vi "Obtain Request Events.vi"(8 "error in":errorcluster, 10 "Create New? (F)":bool) -> (0 "error out":errorcluster, 2 "DemoData Generator Request Events":T1)   [LabVIEW 2016, in "DemoData Generator.lvlib"]
doc: "This VI Obtains/Creates the Requests events that will be used for other modules to communicate with the module that owns this VI. These Requests events will be accessed only via Public API methods for this module.\n\n<b>NOTE</b>: The contents of this VI are automatically generated and modified by the <b>Tools > DQMH Consortium > DQMH</b> utilities. Consider using those utilities instead of making your own modifications to this VI.\n_____\nBased on DQMH Project Template 7.0.0.1280."
uses:
  DemoData Generator.lvlib
  Request Events--cluster.ctl
  Stop Argument--cluster.ctl
  Show Panel Argument--cluster.ctl
  Hide Panel Argument--cluster.ctl
  Get Module Execution Status Argument--cluster.ctl
  Show Diagram Argument--cluster.ctl
  Wake-Up Data Reader Argument--cluster.ctl
  Sleep Data Reader Argument--cluster.ctl
  Start Demo Data Argument--cluster.ctl
  Stop Demo Data Argument--cluster.ctl
panel:
  # "NOTE: The contents of this VI are automatically generated and modified by the Tools > DQMH Consortium > DQMH utilities. Consider using those utilities instead of making your own modifications to this VI."
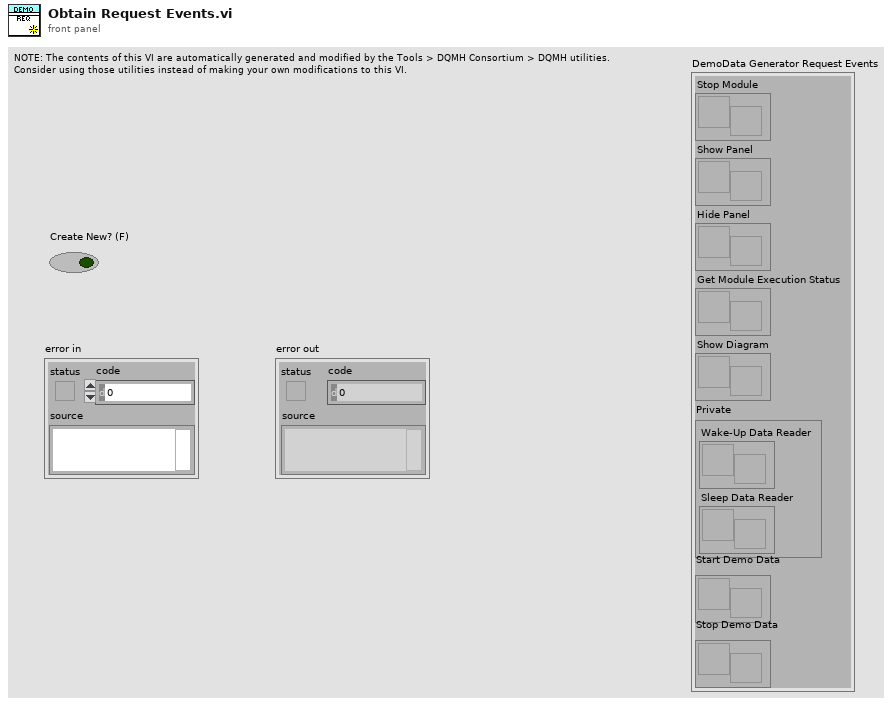
[diagram p1: front panel]
types:
  T1 = typedef "DemoData Generator.lvlib/Request Events--cluster.ctl" = cluster{"Stop Module":refnum<user-event>, "Show Panel":refnum<user-event>, "Hide Panel":refnum<user-event>, "Get Module Execution Status":refnum<user-event>, "Show Diagram":refnum<user-event>, "Private":cluster{"Wake-Up Data Reader":refnum<user-event>, "Sleep Data Reader":refnum<user-event>}, "Start Demo Data":refnum<user-event>, "Stop Demo Data":refnum<user-event>}
  T2 = typedef "DemoData Generator.lvlib/Stop Demo Data Argument--cluster.ctl" = cluster{"Boolean":bool}
  T3 = typedef "DemoData Generator.lvlib/Start Demo Data Argument--cluster.ctl" = cluster{"Boolean":bool}
  T4 = typedef "DemoData Generator.lvlib/Sleep Data Reader Argument--cluster.ctl" = cluster{"Boolean":bool}
  T5 = typedef "DemoData Generator.lvlib/Wake-Up Data Reader Argument--cluster.ctl" = cluster{"Boolean":bool, "Data File.file path":path}
  T6 = typedef "DemoData Generator.lvlib/Hide Panel Argument--cluster.ctl" = cluster{"Hide Panel?":bool}
  T7 = typedef "DemoData Generator.lvlib/Show Panel Argument--cluster.ctl" = cluster{"Show Panel?":bool}
  T8 = typedef "DemoData Generator.lvlib/Show Diagram Argument--cluster.ctl" = cluster{"Debug?":bool}
  T9 = typedef "DemoData Generator.lvlib/Get Module Execution Status Argument--cluster.ctl" = cluster{"Running?":bool}
  T10 = typedef "DemoData Generator.lvlib/Stop Argument--cluster.ctl" = cluster{"Origin":string, "Exit via Stop Module Req?":bool, "Wait for Module to stop?":bool}
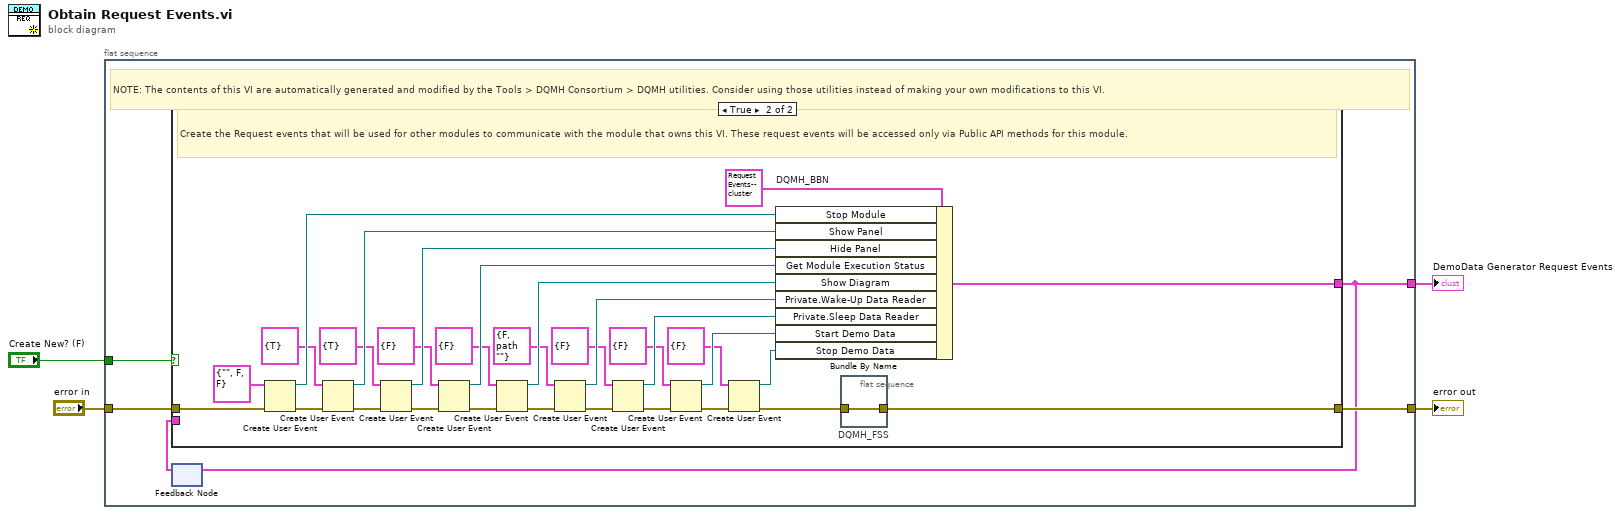
[diagram p0: block diagram]
diagram:
  n1 = flat-sequence {
    tunnel: [w9] -> w4
    tunnel: "error in" -> [w8]
    tunnel: [w6] -> w2
    tunnel: "Create New? (F)" -> [w5]
    frame #0 {
      # "NOTE: The contents of this VI are automatically generated and modified by the Tools > DQMH Consortium > DQMH utilities. Consider using those utilities instead of making your own modifications to this VI."
      n2 = feedback #1() -> (w7:T1)  [unwired: 1 in]
      n3 = case shown="True" w5 {
        tunnel: [w10 w32] -> w9
        tunnel: w8 -> [w10 w42]
        tunnel: [w11 w39] -> w6
        tunnel: w7 -> [w11 _]
        frame False {
          # "Obtain the Request events that were created in a previous call to this VI."
        }
        frame True {
          # "Create the Request events that will be used for other modules to communicate with the module that owns this VI. These request events will be accessed only via Public API methods for this module."
          n4 = Create User Event(user event datatype=T10 {"Origin"="", "Exit via Stop Module Req?"=FALSE, "Wait for Module to stop?"=FALSE} ("Stop Argument"), error in=w42) -> (user event=w40:refnum<user-event>, error out=w37:errorcluster)
          n5 = Create User Event(user event datatype=T7 {"Show Panel?"=TRUE} ("Show Panel Argument"), error in=w37) -> (user event=w36:refnum<user-event>, error out=w35:errorcluster)
          n6 = Create User Event(user event datatype=T6 {"Hide Panel?"=TRUE} ("Hide Panel Argument"), error in=w35) -> (user event=w34:refnum<user-event>, error out=w33:errorcluster)
          n7 = Create User Event(user event datatype=T9 {"Running?"=FALSE} ("Get Module Execution Status Argument"), error in=w33) -> (user event=w30:refnum<user-event>, error out=w31:errorcluster)
          n8 = Create User Event(user event datatype=T8 {"Debug?"=FALSE} ("Show Diagram Argument"), error in=w31) -> (user event=w27:refnum<user-event>, error out=w28:errorcluster)
          n9 = Create User Event(user event datatype=T5 {"Boolean"=FALSE, "Data File.file path"=path ""} ("Wake-Up Data Reader Argument"), error in=w28) -> (user event=w22:refnum<user-event>, error out=w23:errorcluster)
          n10 = Create User Event(user event datatype=T4 {"Boolean"=FALSE} ("Sleep Data Reader Argument"), error in=w23) -> (user event=w19:refnum<user-event>, error out=w20:errorcluster)
          n11 = Create User Event(user event datatype=T3 {"Boolean"=FALSE} ("Start Demo Data Argument"), error in=w20) -> (user event=w16:refnum<user-event>, error out=w17:errorcluster)
          n12 = Create User Event(user event datatype=T2 {"Boolean"=FALSE} ("Stop Demo Data Argument"), error in=w17) -> (user event=w13:refnum<user-event>, error out=w14:errorcluster)
          n13 = Bundle By Name "DQMH_BBN"(cluster=T1 {"Stop Module"=refnum, "Show Panel"=refnum, "Hide Panel"=refnum, "Get Module Execution Status"=refnum, "Show Diagram"=refnum, "Private"={"Wake-Up Data Reader"=refnum, "Sleep Data Reader"=refnum}, "Start Demo Data"=refnum, "Stop Demo Data"=refnum} ("output cluster"), "Stop Module"=w40, "Show Panel"=w36, "Hide Panel"=w34, "Get Module Execution Status"=w30, "Show Diagram"=w27, "Private.Wake-Up Data Reader"=w22, "Private.Sleep Data Reader"=w19, "Start Demo Data"=w16, "Stop Demo Data"=w13) -> (w39:T1)
          n14 = flat-sequence "DQMH_FSS" {
            tunnel: w14 -> [w43]
            tunnel: [w43] -> w32
            frame #0 {
            }
          }
        }
      }
      n15 = feedback-in #1(w6) -> ()
    }
  }
  "DemoData Generator Request Events" <- w2
  "error out" <- w4
